vi "Default Instrument Setup.vi"(8 "error in (no error)":errorcluster, 11 "VISA resource name":refnum<visa-resource-name>) -> (0 "error out":errorcluster, 3 "VISA resource name out":refnum<visa-resource-name>)   [LabVIEW 2012, in "Micos_uic.lvlib"]
doc: "This Utility VI sends a default command string to the instrument whenever a new VISA session is opened, or the instrument is reset. Use this VI as a subVI for the Initialize and Reset VIs. Altering this VI could cause these two VIs to operate incorrectly."
uses:
  Micos_uic.lvlib
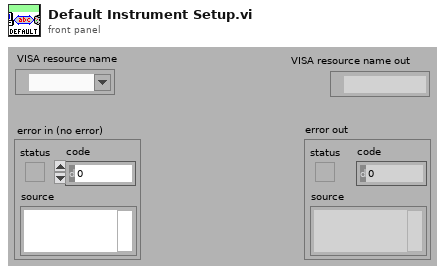
[diagram p1: front panel]
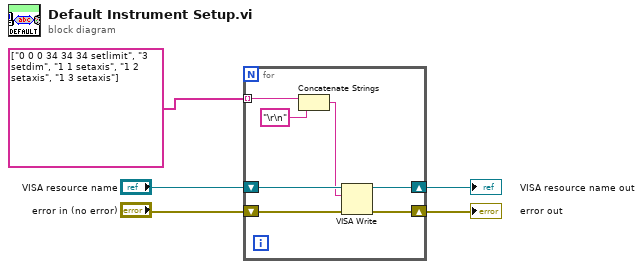
[diagram p0: block diagram]
diagram:
  n1 = for {
    tunnel: string[] ["0 0 0 34 34 34 setlimit", "3 setdim", "1 1 setaxis", "1 2 setaxis", "1 3 setaxis"] -> [w8] mode=indexing
    shift-right: [w10] -> w3
    shift-left: "VISA resource name" -> [w12]
    shift-right: [w9] -> w2
    shift-left: "error in (no error)" -> [w11]
    n2 = Concatenate Strings(w8, "\r\n" ("string")) -> (w7:string)
    n3 = VISA Write(VISA resource name=w12, write buffer=w7, error in (no error)=w11) -> (VISA resource name out=w10:refnum<visa-resource-name>, error out=w9:errorcluster)  [unwired: 1 out]
  }
  "error out" <- w2
  "VISA resource name out" <- w3
